vi "Receiver_Example - 2 Channel - Experiment_10.vi"() -> ()   [LabVIEW 2022 SP3]
uses:
  <vilib>/httpClient/LabVIEWHTTPClient.lvlib
panel:
  out "LP - CH0 3":dbl format="%#_4g"
  out "LP - CH0 2":dbl format="%#_4g"
  out "HP - CH0 3":dbl format="%#_4g"
  out "HP - CH0 2":dbl format="%#_4g"
  out ".not. x?":bool
  out "BER 16QAM":dbl
  out "LP - CH0":dbl format="%#_4g"
  in  "url 2":string="http://Cobot280-02.local:5000"
  out "Numeric":i32
  out "HP - CH0":dbl format="%#_4g"
  in  "url":string="http://Cobot280-01.local:5000"
  out "x = 0?":bool
  out "iterationsIM":dbl
  in  "State":i32
  in  "Counter":dbl
  in  "OFDM - 4QAM/16QAM":bool
  in  "Tab Control 3":enum32{"OFDM - 4QAM", "16QAM"}(tab)
  in  "Tab Control":enum32{"USRP Parameters", "Rx Info", "BER"}(tab)
  in  "USRP ControledParameters":T1={"Active Antenna"="RX2", "Gain (dB)"=10.0, "Carrier Frequency"=2400000000.0, "IQ Rate"=2000000.0, "Active channels"="0,1"} {"IQ Rate" format="%#_6p"; "Carrier Frequency" format="%#_6p"; "Gain (dB)" format="%#_6f"}
  in  "Device selection":refnum<k15>="RIO0"
  in  "Trigger level":dbl=0.005 format="%f"
  out "CH0":T2
  out "CH1":T2
  out "SIG valid? - CH1":bool
  out "SIG valid? - CH0":bool
  out "Frequency offset - CH1":dbl
  out "Frequency offset - CH0":dbl
  out "Coerced Parameters":T3={"IQ Rate"=100000.0, "Carrier  Freq."=100000.0, "Gain"=0.0} {"Gain" format="%#_6f"; "Carrier  Freq." format="%#_6p"; "IQ Rate" format="%#_6p"}
  out "Error out":errorcluster
  in  "Expected message LP - CH0":string="Non Critical Data\nNon Critical Data\nNon Critical Data\nNon Critical Data\nNon Critical Data"
  in  "Expected message - CH1":string="Critical Dataaaaa\nCritical Dataaaaa\nCritical Dataaaaa\nCritical Dataaaaa\nCritical Dataaaaa"
  out "Expected message LP Detected CH0":string="Non Critical Data\nNon Critical Data\nNon Critical Data\nNon Critical Data\nNon Critical Data"
  out "Expected message HP Detected CH1":string="Non Critical Data\nNon Critical Data\nNon Critical Data\nNon Critical Data\nNon Critical Data"
  in  "Boolean":bool
  in  "Boolean 3":bool
  out "Expected message HP Detected CH0":string="Non Critical Data\nNon Critical Data\nNon Critical Data\nNon Critical Data\nNon Critical Data"
  in  "Expected message HP - CH0":string="Critical Dataaaaa\nCritical Dataaaaa\nCritical Dataaaaa\nCritical Dataaaaa\nCritical Dataaaaa"
  in  "Boolean 2":bool
  out "Inst. BER HP - CH0":dbl format="%#_4g"
  out "Acc. BER HP - CH0":dbl format="%#_4g"
  out "Acum. Err HP - CH0":dbl
  out "No. Bits HP - CH0":dbl
  out "Acc. BER LP - CH0":dbl format="%#_4g"
  out "Inst. BER - CH1":dbl format="%#_4g"
  out "Inst. BER LP - CH0":dbl format="%#_4g"
  out "No. Bits - CH1":dbl
  out "No. Bits LP - CH0":dbl
  out "Acum. Err - CH1":dbl
  out "Acum. Err LP - CH0":dbl
  in  "Record BER":bool
  in  "Refresh Button":bool
  out "Acc. BER - CH1":dbl format="%#_4g"
  in  "Low-Power Window Size - CH0":dbl=15.0 format="%#_6p"
  in  "High-Power Window Size":dbl=15.0 format="%#_6p"
  in  "Tab Control 2":enum32{"1 Channel", "2 Channel"}(tab)
  in  "Save data 1 channel":bool
  out "Constellation Map 1 Channel":cdb[](graph)
  out "Low-Power BER - 1 Channel":dbl(graph)
  out "High-Power BER - 1 Channel":dbl(graph)
  out "High-Power Decoded message - 1 Channel":string
  out "Low-Power Decoded message - 1 Channel":string
  in  "Color Box":u32(colorbox)=11025761
  in  "Color Box 2":u32(colorbox)=7377308
  out "Low-Power Decoded message - CH0":string
  out "Decoded message - CH1":string
  out "Constellation Map 2 Channel":cluster{"Constellation":cdb[]}[](graph)
  out "Low-Power BER - CH0":dbl(graph)
  out "High-Power BER":T4(graph)
  out "High-Power Decoded message - CH0":string
  out "CH1 2":bool
  out "CH0 2":bool
  in  "Save data 2 channels":bool
  in  "Channel":bool
  in  "Threshold":dbl=10.0
  in  "Save data":bool
  out "Expected message  HP  Detected 2":string="Critical Dataaaaa\nCritical Dataaaaa\nCritical Dataaaaa\nCritical Dataaaaa\nCritical Dataaaaa"
  in  "Boolean 4":bool
  in  "High-Power Window Size 2":dbl=15.0 format="%#_6p"
  out "High-Power Instantaneous BER Graph 2":u8(slide) scale=0.0..100.0
  out "High-Power BER Graph 2":dbl(graph)
  out "No. Bits HP 2":dbl
  out "Acc. BER  HP 2":dbl format="%#_4g"
  out "Acum. Err HP 2":dbl
  out "Inst. BER HP 2":dbl format="%#_4g"
  in  "Expected message 2 HP 2":string="Critical Dataaaaa\nCritical Dataaaaa\nCritical Dataaaaa\nCritical Dataaaaa\nCritical Dataaaaa"
  out "High-Power Decoded Message 2":string
  in  "Record BER 2":bool
  out "Constellation Map 2":cdb[](graph)
  out "Frequency offset 2":dbl
  out "SIG valid? 2":bool
  in  "Refresh Button 2":bool
  out "Error out 2":errorcluster
  in  "error in (no error)":errorcluster
  # "OFDM Superposition Coded Receiver"
  # "1 Channel"
  # "2 Channel"
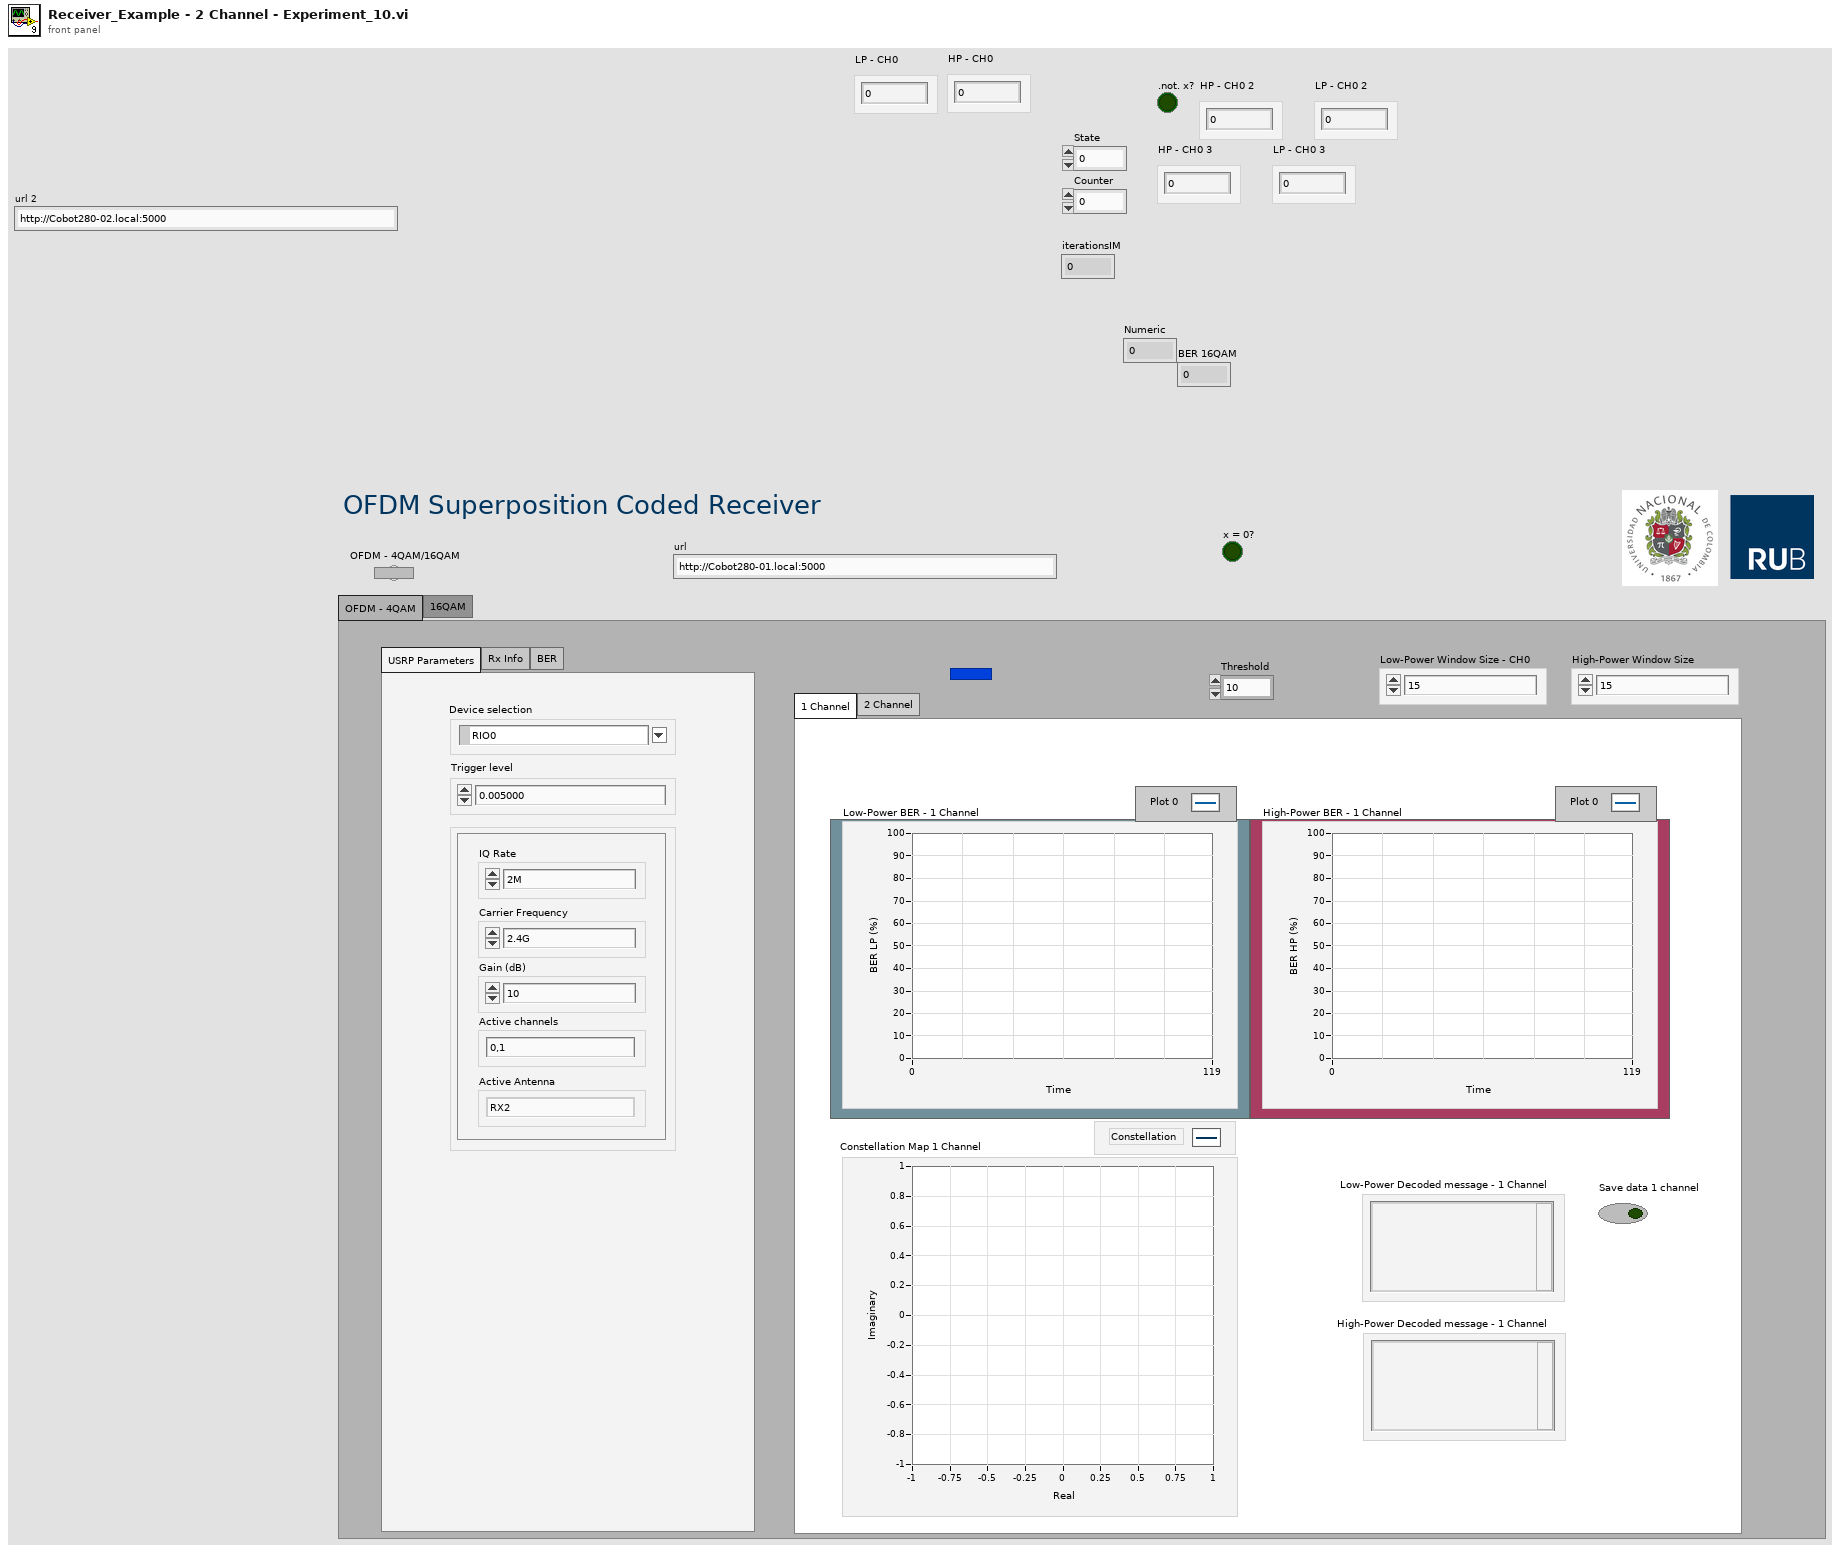
[diagram p1: front panel]
types:
  T1 = cluster{"Active Antenna":string, "Gain (dB)":dbl, "Carrier Frequency":dbl, "IQ Rate":dbl, "Active channels":string}
  T2 = cluster{"Modulation type":enum16{"QPSK(4QAM)", "64QAM", "16QAM", "BPSK"}, "BCC rate (k/n)":enum16{"1/2", "2/3", "3/4"}}
  T3 = cluster{"IQ Rate":dbl, "Carrier  Freq.":dbl, "Gain":dbl}
  T4 = cluster{"Graph Instantaneous BER":dbl, "Graph Instantaneous BER":dbl, "Inst. BER - CH1":dbl}
  T5 = enum16{"open", "replace", "create", "open or create", "replace or create", "replace or create with confirmation"}
  T6 = cluster{"coerced IQ rate":dbl, "coerced carrier frequency":dbl, "coerced gain":dbl}
  T7 = cluster{"Graph Instantaneous BER":dbl, "Graph Instantaneous BER":dbl, "Graph Instantaneous BER":dbl}
  T8 = typedef "LabVIEWHTTPClient.lvlib/ClientHandle.ctl" = refnum<k1>
  T9 = typedef "angle_speed_def.ctl" = cluster{"degrees":dbl[], "speed":i32}
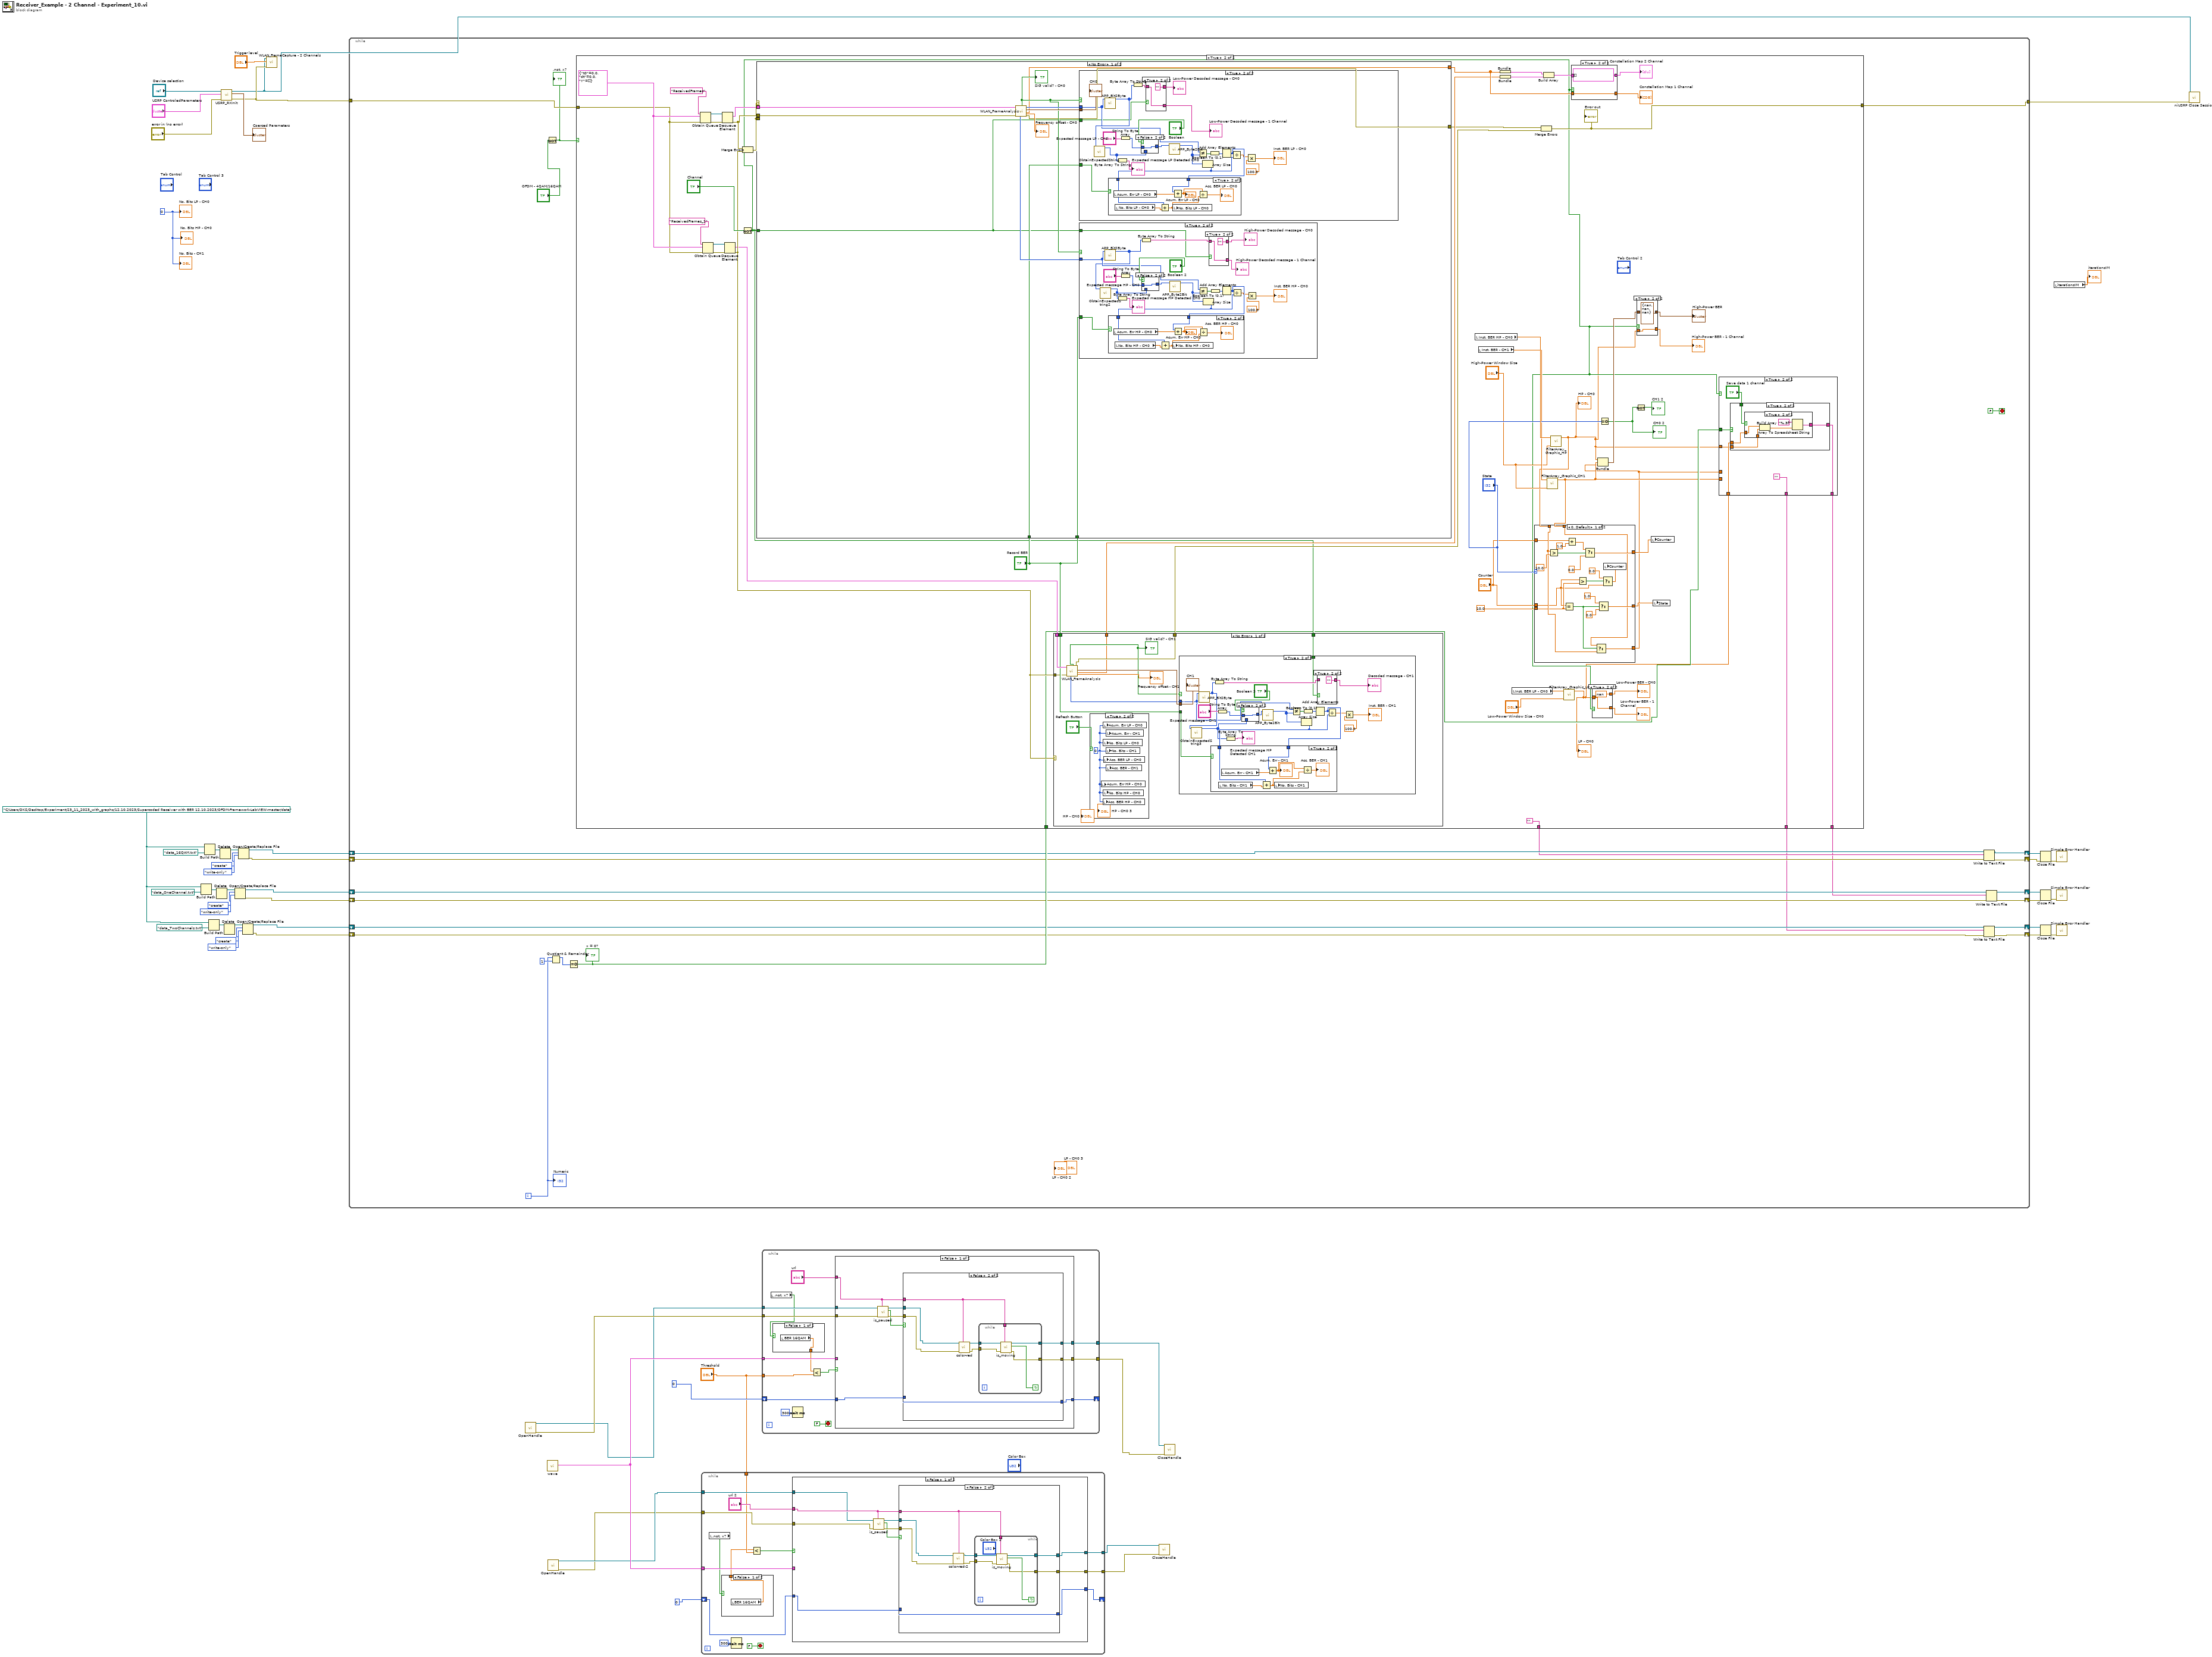
[diagram p0: block diagram]
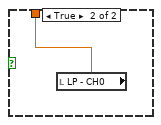
[diagram p2: hidden frame]
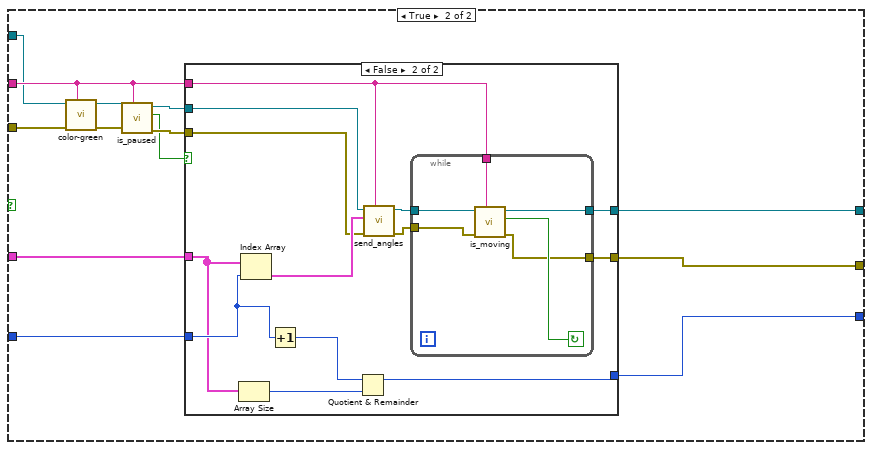
[diagram p4: hidden frame]
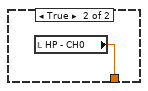
[diagram p6: hidden frame]
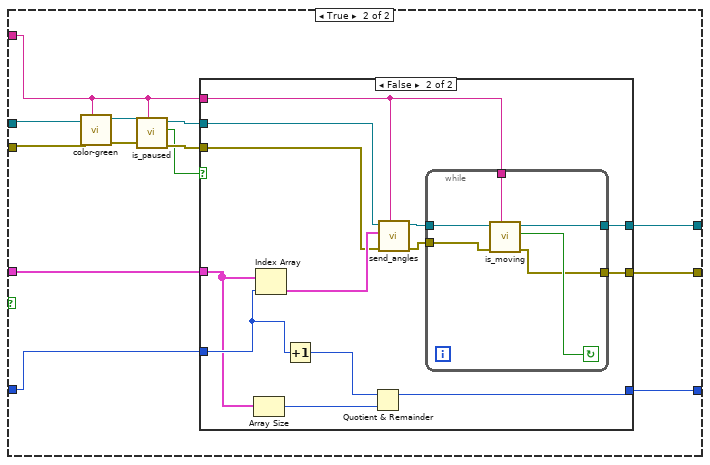
[diagram p8: hidden frame]
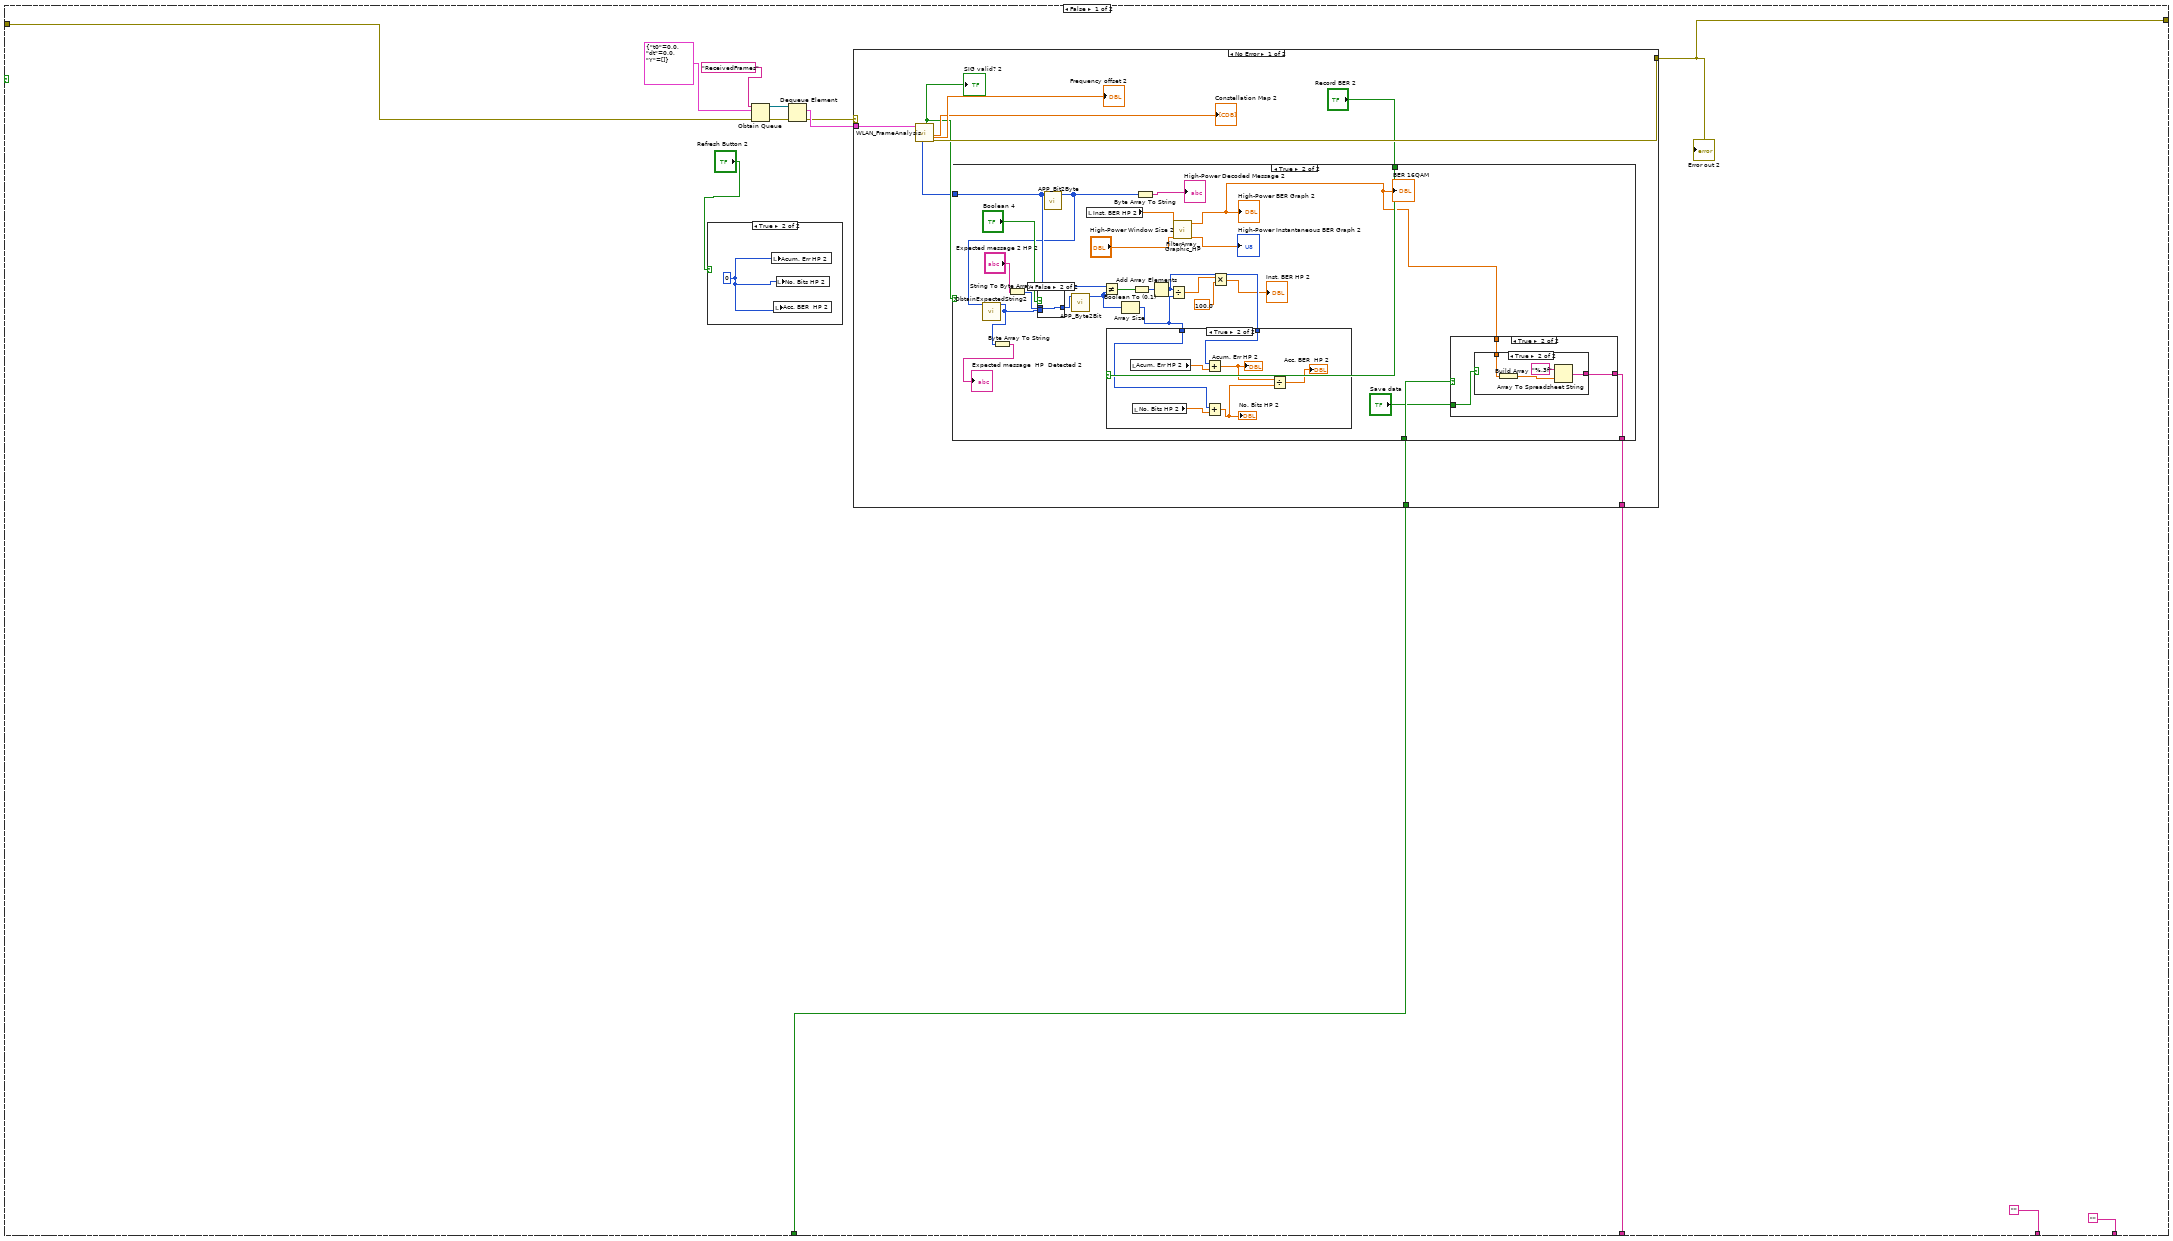
[diagram p10: hidden frame]
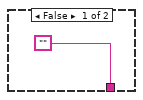
[diagram p12: hidden frame]
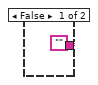
[diagram p13: hidden frame]
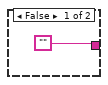
[diagram p14: hidden frame]
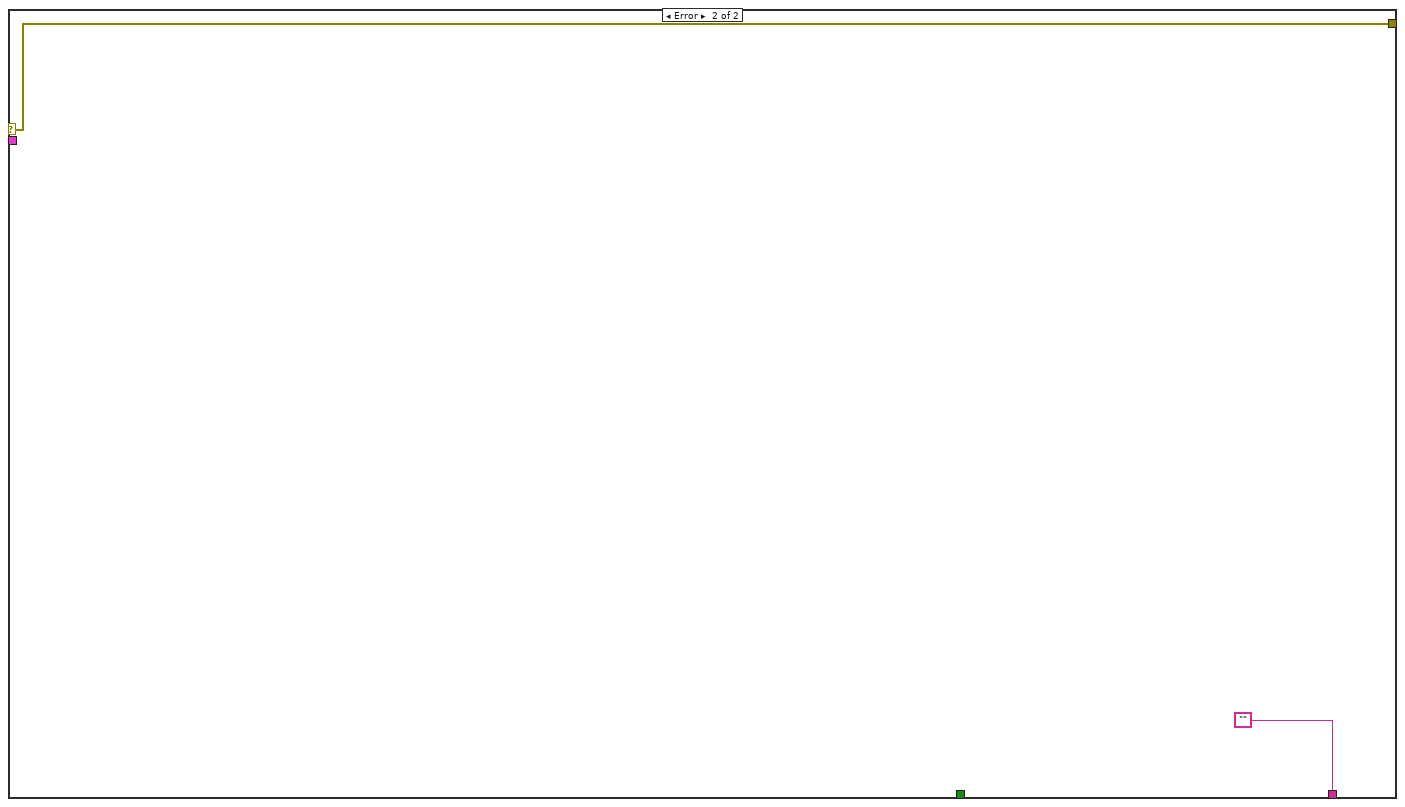
[diagram p17: hidden frame]
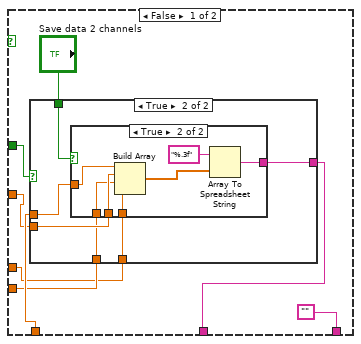
[diagram p18: hidden frame]
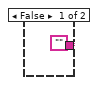
[diagram p19: hidden frame]
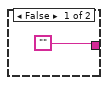
[diagram p20: hidden frame]
diagram:
  w23 = path "C:/Users/DKS/Desktop/Experiment/23_11_2023_with_graphs/12.10.2023/Supercoded Receiver with BER 12.10.2023/OFDM-Framework-LabVIEW-master/data"
  w45 = 0
  n1 = Build Path(base path=w23, name or relative path=path "data_OneChannel.txt" ("default name")) -> (appended path=w33:path)
  n2 = Build Path(base path=w23, name or relative path=path "data_16QAM.txt" ("default name")) -> (appended path=w43:path)
  n3 = Build Path(base path=w23, name or relative path=path "data_TwoChannels.txt" ("default name")) -> (appended path=w28:path)
  n4 = Delete(path (use dialog)=w33) -> (deleted path=w32:path)  [unwired: 4 in, 2 out]
  n5 = Delete(path (use dialog)=w43) -> (deleted path=w42:path)  [unwired: 4 in, 2 out]
  n6 = call "USRP_RXInit.vi"("device names"="Device selection", "USRP ControledParameters"="USRP ControledParameters", "error in (no error)"="error in (no error)") -> ("session handle out"=w48:refnum<k15>, "USRP CoercedParamters"=→"Coerced Parameters":T6, "error out"=w51:errorcluster)  [unwired: 5 in]
  n7 = Delete(path (use dialog)=w28) -> (deleted path=w27:path)  [unwired: 4 in, 2 out]
  n8 = Open/Create/Replace File(file path (use dialog)=w32, operation (0:open)=T5."create", access (0:read/write)=enum16{"read/write", "read-only", "write-only"}."write-only") -> (refnum out=w20:refnum<file>, error out=w19:errorcluster)  [unwired: 1 in, 3 out]
  n9 = Open/Create/Replace File(file path (use dialog)=w42, operation (0:open)=T5."create", access (0:read/write)=enum16{"read/write", "read-only", "write-only"}."write-only") -> (refnum out=w36:refnum<file>, error out=w37:errorcluster)  [unwired: 1 in, 3 out]
  n10 = Open/Create/Replace File(file path (use dialog)=w27, operation (0:open)=T5."create", access (0:read/write)=enum16{"read/write", "read-only", "write-only"}."write-only") -> (refnum out=w18:refnum<file>, error out=w17:errorcluster)  [unwired: 1 in, 3 out]
  n11 = call "WLAN_FrameCapture - 2 Channels.vi"("error in (no error)"=w51, "Trigger level"="Trigger level", "session handle"=w48) -> ()  [unwired: 8 in]
  n12 = while {
    tunnel: w51 -> [w77]
    tunnel: [w76] -> w49
    shift-right: [w69] -> w35
    shift-left: w37 -> [w67]
    shift-right: [w68] -> w34
    shift-left: w36 -> [w66]
    shift-right: [w63] -> w16
    shift-left: w20 -> [w64]
    shift-right: [w61] -> w15
    shift-left: w19 -> [w62]
    shift-right: [w57] -> w14
    shift-left: w18 -> [w60]
    shift-right: [w58] -> w13
    shift-left: w17 -> [w59]
    i -> [w54]
    stop <- FALSE stop-if-true
    n13 = Not(x="OFDM - 4QAM/16QAM") -> (.not. x?=w74:bool)
    ".not. x?" <- w74
    n14 = Quotient & Remainder(x=w54, y=1) -> (x-y*floor(x/y)=w71:i32)  [unwired: 1 out]
    n15 = Equal To 0?(x=w71) -> (x = 0?=w70:bool)
    "x = 0?" <- w70
    n16 = case shown="True" w74 {
      tunnel: w77 -> [w83 w161]
      tunnel: [w82 w160] -> w76
      tunnel: w70 -> [w81 w153]
      tunnel: [w80 ""] -> w65
      tunnel: ["" w152] -> w56
      tunnel: ["" w150] -> w55
      frame False {
        n17 = case shown="True" "Refresh Button 2" {
          frame False {
          }
          frame True {
            w91 = 0
            n18 = local write "Acum. Err HP 2"(w91) -> ()
            n19 = local write "Acc. BER  HP 2"(w91) -> ()
            n20 = local write "No. Bits HP 2"(w91) -> ()
          }
        }
        n21 = Obtain Queue(name (unnamed)="ReceivedFrames", element data type=cluster{"t0":dbl, "dt":dbl, "Y":cdb[]} {"t0"=0.0, "dt"=0.0, "Y"=[]} ("data"), error in (no error)=w83) -> (queue out=w84:refnum<queue>, error out=w87:errorcluster)  [unwired: 2 in, 1 out]
        n22 = Dequeue Element(queue=w84, error in (no error)=w87) -> (element=w86:cluster{"t0":dbl, "dt":dbl, "Y":cdb[]}, error out=w85:errorcluster)  [unwired: 1 in, 2 out]
        n23 = case shown="No Error" w85 {
          selector: w85 -> [_ w146]
          tunnel: w86 -> [w99 _]
          tunnel: [w100 w146] -> w82
          tunnel: w81 -> [w93 _]
          tunnel: [w92 ""] -> w80
          frame No Error {
            n24 = call "WLAN_FrameAnalysis.vi"("input cluster"=w99) -> ("error out"=w100:errorcluster, "Constellation"=→"Constellation Map 2":cdb[], "Frequency offset"=→"Frequency offset 2":dbl, "SIG valid?"=w95:bool, "outputbitsHP"=w94:i8[])  [unwired: 4 in, 2 out]
            "SIG valid? 2" <- w95
            n25 = case shown="True" w95 {
              tunnel: "Record BER 2" -> [_ w120]
              tunnel: w94 -> [_ w115]
              tunnel: w93 -> [_ w105]
              tunnel: ["" w103] -> w92
              frame False {
              }
              frame True {
                n26 = String To Byte Array(string="Expected message 2 HP 2") -> (unsigned byte array=w113:u8[])
                n27 = call "APP_Bit2Byte.vi"("input bit stream"=w115) -> ("output byte stream"=w109:u8[])  [unwired: 10 in]
                n28 = call "ObtainExpectedString2.vi"("Array"=w109) -> ("detectedMessage"=w111:i8[])  [unwired: 9 in]
                n29 = Byte Array To String(unsigned byte array=w111) -> (string=→"Expected message  HP  Detected 2":string)
                n30 = case shown="False" "Boolean 4" {
                  tunnel: [w136 w137] -> w114
                  tunnel: w113 -> [_ w137]
                  tunnel: w111 -> [w136 _]
                  frame True {
                  }
                  frame False {
                  }
                }
                n31 = call "APP_Byte2Bit.vi"("input byte stream"=w114) -> ("output bit stream"=w116:i8[])  [unwired: 10 in]
                n32 = local read "Inst. BER HP 2"() -> (w119:dbl)
                n33 = Not Equal?(x=w115, y=w116) -> (x != y?=w124:bool[])
                n34 = Array Size(array=w116) -> (size(s)=w121:i32)
                n35 = Boolean To (0,1)(Boolean=w124) -> (0, 1=w123:i16[])
                n36 = Byte Array To String(unsigned byte array=w109) -> (string=→"High-Power Decoded Message 2":string)
                n37 = Add Array Elements(numeric array=w123) -> (sum=w122:i16)
                n38 = case shown="True" w120 {
                  tunnel: w122 -> [_ w143]
                  tunnel: w121 -> [_ w138]
                  frame False {
                  }
                  frame True {
                    n39 = local read "Acum. Err HP 2"() -> (w144:dbl)
                    n40 = local read "No. Bits HP 2"() -> (w140:dbl)
                    n41 = Add(x=w143, y=w144) -> (x+y=w142:dbl)
                    "Acum. Err HP 2" <- w142
                    n42 = Add(x=w138, y=w140) -> (x+y=w139:dbl)
                    "No. Bits HP 2" <- w139
                    n43 = Divide(x=w142, y=w139) -> (x/y=→"Acc. BER  HP 2":dbl)
                  }
                }
                n44 = Divide(x=w122, y=w121) -> (x/y=w108:dbl)
                n45 = call "FilterArray_Graphic_HP.vi"("Window Size"="High-Power Window Size 2", "Instantaneous BER"=w119) -> ("Slide Bar"=→"High-Power Instantaneous BER Graph 2":dbl, "Graph Instantaneous BER"=w102:dbl)  [unwired: 4 in]
                "High-Power BER Graph 2" <- w102
                "BER 16QAM" <- w102
                n46 = Multiply(x=w108, y=100.0) -> (x*y=→"Inst. BER HP 2":dbl)
                n47 = case shown="True" w105 {
                  tunnel: ["" w130] -> w103
                  tunnel: w102 -> [_ w129]
                  tunnel: "Save data" -> [_ w128]
                  frame False {
                  }
                  frame True {
                    n48 = case shown="True" w128 {
                      tunnel: ["" w133] -> w130
                      tunnel: w129 -> [_ w132]
                      frame False {
                      }
                      frame True {
                        n49 = Build Array(w132) -> (w135:dbl[])
                        n50 = Array To Spreadsheet String(array=w135, 3:"%.3f") -> (spreadsheet string=w133:string)  [unwired: 1 out]
                      }
                    }
                  }
                }
              }
            }
          }
          frame Error {
          }
        }
        "Error out 2" <- w82
      }
      frame True {
        w197 = cluster{"t0":dbl, "dt":dbl, "Y":cdb[]} {"t0"=0.0, "dt"=0.0, "Y"=[]} ("data")
        n51 = Obtain Queue(name (unnamed)="ReceivedFrames", element data type=w197, error in (no error)=w161) -> (queue out=w162:refnum<queue>, error out=w164:errorcluster)  [unwired: 2 in, 1 out]
        n52 = Obtain Queue(name (unnamed)="ReceivedFrames_1", element data type=w197, error in (no error)=w161) -> (queue out=w166:refnum<queue>, error out=w167:errorcluster)  [unwired: 2 in, 1 out]
        n53 = Dequeue Element(queue=w162, error in (no error)=w164) -> (element=w163:cluster{"t0":dbl, "dt":dbl, "Y":cdb[]}, error out=w170:errorcluster)  [unwired: 1 in, 2 out]
        n54 = Dequeue Element(queue=w166, error in (no error)=w167) -> (element=w172:cluster{"t0":dbl, "dt":dbl, "Y":cdb[]}, error out=w176:errorcluster)  [unwired: 1 in, 2 out]
        n55 = Not(x="Channel") -> (.not. x?=w154:bool)
        n56 = Merge Errors(w170, w176) -> (w169:errorcluster)
        n57 = case shown="No Error" w169 {
          tunnel: w163 -> [w342 _]
          tunnel: w169 -> [_ w416]
          tunnel: w170 -> [w339 _]
          tunnel: [w338 dbl[] []] -> w188
          tunnel: [w337 w416] -> w173
          tunnel: "Record BER" -> [w336 _]
          tunnel: "Record BER" -> [w335 _]
          tunnel: w154 -> [w334 _]
          frame No Error {
            n58 = call "WLAN_FrameAnalysis.vi"("error in (no error)"=w339, "input cluster"=w342) -> ("error out"=w337:errorcluster, "Constellation"=w338:cdb[], "Modulation parameter"=w343:T2, "output bits"=w344:i8[], "Frequency offset"=→"Frequency offset - CH0":dbl, "SIG valid?"=w340:bool, "outputbitsHP"=w341:i8[])  [unwired: 3 in]
            "SIG valid? - CH0" <- w340
            n59 = case shown="True" w340 {
              tunnel: w344 -> [_ w385]
              tunnel: w343 -> [_ w401]
              tunnel: w335 -> [_ w397]
              tunnel: w334 -> [_ w380]
              frame False {
              }
              frame True {
                n60 = call "APP_Bit2Byte.vi"("input bit stream"=w385) -> ("output byte stream"=w389:u8[])  [unwired: 10 in]
                n61 = call "ObtainExpectedString.vi"("Array"=w389) -> ("detectedMessage"=w386:i8[])  [unwired: 9 in]
                n62 = Byte Array To String(unsigned byte array=w386) -> (string=→"Expected message LP Detected CH0":string)
                n63 = String To Byte Array(string="Expected message LP - CH0") -> (unsigned byte array=w390:u8[])
                n64 = Byte Array To String(unsigned byte array=w389) -> (string=w383:string)
                n65 = case shown="False" "Boolean" {
                  tunnel: [w406 w407] -> w392
                  tunnel: w390 -> [_ w407]
                  tunnel: w386 -> [w406 _]
                  frame True {
                  }
                  frame False {
                  }
                }
                n66 = case shown="True" w380 {
                  tunnel: w383 -> [w403 w405]
                  tunnel: ["" ("string") w405] -> w382
                  tunnel: [w403 "" ("string")] -> w381
                  frame False {
                  }
                  frame True {
                  }
                }
                "Low-Power Decoded message - CH0" <- w381
                "Low-Power Decoded message - 1 Channel" <- w382
                n67 = call "APP_Byte2Bit.vi"("input byte stream"=w392) -> ("output bit stream"=w391:i8[])  [unwired: 10 in]
                n68 = Not Equal?(x=w385, y=w391) -> (x != y?=w399:bool[])
                n69 = Array Size(array=w391) -> (size(s)=w396:i32)
                n70 = Boolean To (0,1)(Boolean=w399) -> (0, 1=w400:i16[])
                n71 = Add Array Elements(numeric array=w400) -> (sum=w395:i16)
                n72 = case shown="True" w397 {
                  tunnel: w396 -> [_ w413]
                  tunnel: w395 -> [_ w411]
                  frame False {
                  }
                  frame True {
                    n73 = local read "Acum. Err LP - CH0"() -> (w412:dbl)
                    n74 = local read "No. Bits LP - CH0"() -> (w414:dbl)
                    n75 = Add(x=w413, y=w414) -> (x+y=w410:dbl)
                    n76 = Add(x=w411, y=w412) -> (x+y=w409:dbl)
                    "Acum. Err LP - CH0" <- w409
                    n77 = local write "No. Bits LP - CH0"(w410) -> ()
                    n78 = Divide(x=w409, y=w410) -> (x/y=→"Acc. BER LP - CH0":dbl)
                  }
                }
                n79 = Divide(x=w395, y=w396) -> (x/y=w394:dbl)
                n80 = Multiply(x=w394, y=100.0) -> (x*y=→"Inst. BER LP - CH0":dbl)
                "CH0" <- w401
              }
            }
            n81 = case shown="True" w340 {
              tunnel: w341 -> [_ w353]
              tunnel: w336 -> [_ w363]
              tunnel: w334 -> [_ w346]
              frame False {
              }
              frame True {
                n82 = call "APP_Bit2Byte.vi"("input bit stream"=w353) -> ("output byte stream"=w352:u8[])  [unwired: 10 in]
                n83 = call "ObtainExpectedString2.vi"("Array"=w352) -> ("detectedMessage"=w351:i8[])  [unwired: 9 in]
                n84 = Byte Array To String(unsigned byte array=w351) -> (string=→"Expected message HP Detected CH0":string)
                n85 = String To Byte Array(string="Expected message HP - CH0") -> (unsigned byte array=w356:u8[])
                n86 = Byte Array To String(unsigned byte array=w352) -> (string=w347:string)
                n87 = case shown="False" "Boolean 2" {
                  tunnel: [w371 w372] -> w358
                  tunnel: w356 -> [_ w372]
                  tunnel: w351 -> [w371 _]
                  frame True {
                  }
                  frame False {
                  }
                }
                n88 = call "APP_Byte2Bit.vi"("input byte stream"=w358) -> ("output bit stream"=w357:i8[])  [unwired: 10 in]
                n89 = Not Equal?(x=w353, y=w357) -> (x != y?=w365:bool[])
                n90 = Array Size(array=w357) -> (size(s)=w362:i32)
                n91 = case shown="True" w346 {
                  tunnel: w347 -> [w368 w370]
                  tunnel: ["" ("string") w370] -> w348
                  tunnel: [w368 "" ("string")] -> w349
                  frame False {
                  }
                  frame True {
                  }
                }
                "High-Power Decoded message - CH0" <- w349
                "High-Power Decoded message - 1 Channel" <- w348
                n92 = Boolean To (0,1)(Boolean=w365) -> (0, 1=w366:i16[])
                n93 = Add Array Elements(numeric array=w366) -> (sum=w361:i16)
                n94 = case shown="True" w363 {
                  tunnel: w362 -> [_ w378]
                  tunnel: w361 -> [_ w376]
                  frame False {
                  }
                  frame True {
                    n95 = local read "Acum. Err HP - CH0"() -> (w377:dbl)
                    n96 = local read "No. Bits HP - CH0"() -> (w379:dbl)
                    n97 = Add(x=w378, y=w379) -> (x+y=w375:dbl)
                    n98 = local write "No. Bits HP - CH0"(w375) -> ()
                    n99 = Add(x=w376, y=w377) -> (x+y=w374:dbl)
                    "Acum. Err HP - CH0" <- w374
                    n100 = Divide(x=w374, y=w375) -> (x/y=→"Acc. BER HP - CH0":dbl)
                  }
                }
                n101 = Divide(x=w361, y=w362) -> (x/y=w360:dbl)
                n102 = Multiply(x=w360, y=100.0) -> (x*y=→"Inst. BER HP - CH0":dbl)
              }
            }
          }
          frame Error {
          }
        }
        n103 = case shown="No Error" w176 {
          tunnel: w172 -> [w294 _]
          tunnel: "Record BER" -> [w292 _]
          tunnel: [w291 w333] -> w174
          tunnel: [w290 dbl[] []] -> w175
          tunnel: w176 -> [w289 w333]
          tunnel: w154 -> [w288 _]
          frame No Error {
            n104 = call "WLAN_FrameAnalysis.vi"("error in (no error)"=w289, "input cluster"=w294) -> ("error out"=w291:errorcluster, "Constellation"=w290:cdb[], "Modulation parameter"=w297:T2, "Frequency offset"=→"Frequency offset - CH1":dbl, "SIG valid?"=w293:bool, "outputbitsHP"=w295:i8[])  [unwired: 3 in, 1 out]
            "SIG valid? - CH1" <- w293
            n105 = case shown="True" "Refresh Button" {
              frame False {
              }
              frame True {
                w299 = 0
                n106 = local write "Acum. Err HP - CH0"(w299) -> ()
                n107 = local write "Acc. BER HP - CH0"(w299) -> ()
                n108 = local write "Acum. Err LP - CH0"(w299) -> ()
                n109 = local write "No. Bits LP - CH0"(w299) -> ()
                n110 = local write "No. Bits HP - CH0"(w299) -> ()
                n111 = local write "Acc. BER LP - CH0"(w299) -> ()
                n112 = local write "Acum. Err - CH1"(w299) -> ()
                n113 = local write "No. Bits - CH1"(w299) -> ()
                n114 = local write "Acc. BER - CH1"(w299) -> ()
              }
            }
            n115 = case shown="True" w293 {
              tunnel: w295 -> [_ w306]
              tunnel: w297 -> [_ w320]
              tunnel: w292 -> [_ w303]
              tunnel: w288 -> [_ w300]
              frame False {
              }
              frame True {
                n116 = call "APP_Bit2Byte.vi"("input bit stream"=w306) -> ("output byte stream"=w309:u8[])  [unwired: 10 in]
                n117 = call "ObtainExpectedString3.vi"("Array"=w309) -> ("detectedMessage"=w308:i8[])  [unwired: 9 in]
                n118 = Byte Array To String(unsigned byte array=w309) -> (string=w301:string)
                n119 = String To Byte Array(string="Expected message - CH1") -> (unsigned byte array=w310:u8[])
                n120 = Byte Array To String(unsigned byte array=w308) -> (string=→"Expected message HP Detected CH1":string)
                n121 = case shown="False" "Boolean 3" {
                  tunnel: [w323 w324] -> w312
                  tunnel: w310 -> [_ w324]
                  tunnel: w308 -> [w323 _]
                  frame True {
                  }
                  frame False {
                  }
                }
                n122 = call "APP_Byte2Bit.vi"("input byte stream"=w312) -> ("output bit stream"=w311:i8[])  [unwired: 10 in]
                n123 = Not Equal?(x=w306, y=w311) -> (x != y?=w318:bool[])
                n124 = Array Size(array=w311) -> (size(s)=w316:i32)
                n125 = Boolean To (0,1)(Boolean=w318) -> (0, 1=w319:i16[])
                n126 = Add Array Elements(numeric array=w319) -> (sum=w315:i16)
                n127 = case shown="True" w303 {
                  tunnel: w316 -> [_ w330]
                  tunnel: w315 -> [_ w328]
                  frame False {
                  }
                  frame True {
                    n128 = local read "No. Bits - CH1"() -> (w331:dbl)
                    n129 = local read "Acum. Err - CH1"() -> (w329:dbl)
                    n130 = Add(x=w330, y=w331) -> (x+y=w327:dbl)
                    n131 = Add(x=w328, y=w329) -> (x+y=w326:dbl)
                    "Acum. Err - CH1" <- w326
                    n132 = local write "No. Bits - CH1"(w327) -> ()
                    n133 = Divide(x=w326, y=w327) -> (x/y=→"Acc. BER - CH1":dbl)
                  }
                }
                n134 = case shown="True" w300 {
                  tunnel: w301 -> [w321 _]
                  tunnel: [w321 "" ("string")] -> w302
                  frame False {
                  }
                  frame True {
                  }
                }
                "Decoded message - CH1" <- w302
                n135 = Divide(x=w315, y=w316) -> (x/y=w313:dbl)
                n136 = Multiply(x=w313, y=100.0) -> (x*y=→"Inst. BER - CH1":dbl)
                "CH1" <- w320
              }
            }
          }
          frame Error {
          }
        }
        n137 = local read "Inst. BER HP - CH0"() -> (w193:dbl)
        n138 = local read "Inst. BER - CH1"() -> (w183:dbl)
        n139 = Bundle("Constellation"=w188) -> (w187:cluster{"Constellation":cdb[]})  [unwired: 1 in]
        n140 = Bundle("Constellation"=w175) -> (w171:cluster{"Constellation":cdb[]})  [unwired: 1 in]
        n141 = local read "Inst. BER LP - CH0"() -> (w156:dbl)
        n142 = Merge Errors(w173, w174) -> (w160:errorcluster)
        "Error out" <- w160
        n143 = Build Array(w187, w171) -> (w190:cluster{"Constellation":cdb[]}[])
        n144 = call "FilterArray_Graphic_CH1.vi"("Window Size"="High-Power Window Size", "Instantaneous BER"=w183) -> ("Graph Instantaneous BER"=w151:dbl)  [unwired: 4 in, 1 out]
        n145 = call "FilterArray_Graphic_HP.vi"("Window Size"="High-Power Window Size", "Instantaneous BER"=w193) -> ("Graph Instantaneous BER"=w148:dbl)  [unwired: 4 in, 1 out]
        "HP - CH0" <- w148
        n146 = case shown="0, Default" "State" {
          tunnel: "Counter" -> [w256 w276]
          tunnel: [w263 w279] -> w179
          tunnel: "Counter" -> [w251 w269]
          tunnel: [w260 w278] -> w180
          tunnel: [w258 w277] -> w149
          tunnel: w148 -> [w257 w274]
          tunnel: w151 -> [w255 w275]
          tunnel: 10.0 ("y") -> [w254 w270]
          frame 0, Default {
            n147 = Greater?(x=w257, y=10.0) -> (0:w264:bool)
            n148 = Equal?(x=w251, y=w254) -> (x = y?=w259:bool)
            n149 = Add(x=w256, y=1.0) -> (x+y=w266:dbl)
            n150 = Greater?(x=w251, y=w254) -> (0:w253:bool)
            n151 = Select(t=w266, s=w264, f=0.0) -> (s? t:f=w263:dbl)
            n152 = Select(t=w255, s=w259, f=w257) -> (s? t:f=w258:dbl)
            n153 = Select(t=1.0, s=w259, f=0.0) -> (s? t:f=w260:dbl)
            n154 = Select(t=0.0, s=w253, f=w251) -> (s? t:f=w250:dbl)
            n155 = local write "Counter"(w250) -> ()
          }
          frame 1 {
            n156 = Less?(x=w274, y=10.0) -> (x < y?=w280:bool)
            n157 = Greater?(x=w269, y=w270) -> (0:w272:bool)
            n158 = Equal?(x=w269, y=w270) -> (x = y?=w282:bool)
            n159 = Add(x=w276, y=1.0) -> (x+y=w286:dbl)
            n160 = Select(t=w286, s=w280, f=0.0) -> (s? t:f=w279:dbl)
            n161 = Select(t=0.0, s=w272, f=w269) -> (s? t:f=w273:dbl)
            n162 = local write "Counter"(w273) -> ()
            n163 = Select(t=w274, s=w282, f=w275) -> (s? t:f=w277:dbl)
            n164 = Select(t=0.0, s=w282, f=1.0) -> (s? t:f=w278:dbl)
          }
        }
        n165 = call "FilterArray_Graphic_LP.vi"("Window Size"="Low-Power Window Size - CH0", "Instantaneous BER"=w156) -> ("Graph Instantaneous BER"=w147:dbl)  [unwired: 4 in, 1 out]
        "LP - CH0" <- w147
        n166 = case shown="True" w154 {
          tunnel: [cdb[] [] ("Constellation") w249] -> w189
          tunnel: w188 -> [_ w249]
          tunnel: w190 -> [w247 _]
          tunnel: [w247 cluster{"Constellation":cdb[]}[] []] -> w191
          frame False {
          }
          frame True {
          }
        }
        "Constellation Map 2 Channel" <- w191
        "Constellation Map 1 Channel" <- w189
        n167 = case shown="True" w154 {
          tunnel: w147 -> [w239 w241]
          tunnel: [nan ("Graph Instantaneous BER") w241] -> w157
          tunnel: [w239 nan ("Graph Instantaneous BER")] -> w158
          frame False {
          }
          frame True {
          }
        }
        "Low-Power BER - CH0" <- w158
        "Low-Power BER - 1 Channel" <- w157
        n168 = Bundle("Graph Instantaneous BER"=w148, "Graph Instantaneous BER"=w151, "Graph Instantaneous BER"=w149) -> (w195:T7)  [unwired: 1 in]
        n169 = Equal To 0?(x="State") -> (x = 0?=w186:bool)
        "CH0 2" <- w186
        n170 = Not(x=w186) -> (.not. x?=→"CH1 2":bool)
        n171 = case shown="True" w154 {
          tunnel: w148 -> [_ w245]
          tunnel: [nan w245] -> w194
          tunnel: w195 -> [w243 _]
          tunnel: [w243 T7 {"Graph Instantaneous BER"=nan, "Graph Instantaneous BER"=nan, "Graph Instantaneous BER"=nan}] -> w196
          frame False {
          }
          frame True {
          }
        }
        "High-Power BER" <- w196
        "High-Power BER - 1 Channel" <- w194
        n172 = local write "Counter"(w179) -> ()
        n173 = local write "State"(w180) -> ()
        n174 = case shown="True" w154 {
          tunnel: w147 -> [w202 w226]
          tunnel: w148 -> [w201 w225]
          tunnel: w153 -> [w204 w224]
          tunnel: ["" w222] -> w152
          tunnel: w151 -> [w200 _]
          tunnel: w149 -> [w199 _]
          tunnel: [w198 ""] -> w150
          frame False {
            n175 = case shown="True" w204 {
              tunnel: ["" w212] -> w198
              tunnel: w202 -> [_ w210]
              tunnel: w201 -> [_ w211]
              tunnel: "Save data 2 channels" -> [_ w209]
              tunnel: w200 -> [_ w208]
              tunnel: w199 -> [_ w207]
              frame False {
              }
              frame True {
                n176 = case shown="True" w209 {
                  tunnel: ["" w218] -> w212
                  tunnel: w210 -> [_ w217]
                  tunnel: w211 -> [_ w216]
                  tunnel: w208 -> [_ w215]
                  tunnel: w207 -> [_ w214]
                  frame False {
                  }
                  frame True {
                    n177 = Build Array(w217, w216, w215, w214) -> (w220:dbl[])
                    n178 = Array To Spreadsheet String(array=w220, 3:"%.3f") -> (spreadsheet string=w218:string)  [unwired: 1 out]
                  }
                }
              }
            }
          }
          frame True {
            n179 = case shown="True" w224 {
              tunnel: ["" w231] -> w222
              tunnel: w226 -> [_ w229]
              tunnel: w225 -> [_ w230]
              tunnel: "Save data 1 channel" -> [_ w228]
              frame False {
              }
              frame True {
                n180 = case shown="True" w228 {
                  tunnel: ["" w235] -> w231
                  tunnel: w229 -> [_ w234]
                  tunnel: w230 -> [_ w233]
                  frame False {
                  }
                  frame True {
                    n181 = Build Array(w234, w233) -> (w237:dbl[])
                    n182 = Array To Spreadsheet String(array=w237, 3:"%.3f") -> (spreadsheet string=w235:string)  [unwired: 1 out]
                  }
                }
              }
            }
          }
        }
      }
    }
    n183 = Write to Text File(file (use dialog)=w60, text=w55, error in=w59) -> (refnum out=w57:refnum<file>, error out=w58:errorcluster)  [unwired: 1 in, 1 out]
    n184 = Write to Text File(file (use dialog)=w66, text=w65, error in=w67) -> (refnum out=w68:refnum<file>, error out=w69:errorcluster)  [unwired: 1 in, 1 out]
    n185 = Write to Text File(file (use dialog)=w64, text=w56, error in=w62) -> (refnum out=w63:refnum<file>, error out=w61:errorcluster)  [unwired: 1 in, 1 out]
    "Numeric" <- w54
  }
  n186 = call <vilib>:"OpenHandle.vi"() -> ("client handle out"=w7:T8, "error out"=w8:errorcluster)  [unwired: 14 in]
  n187 = call "wave.vi"() -> ("sequenz"=w9:T9[])  [unwired: 11 in]
  n188 = call <vilib>:"OpenHandle.vi"() -> ("client handle out"=w3:T8, "error out"=w2:errorcluster)  [unwired: 14 in]
  n189 = while {
    shift-right: [w425] -> _
    shift-left: 0 -> [w426]
    tunnel: w9 -> [w424]
    tunnel: w2 -> [w423]
    tunnel: w3 -> [w422]
    tunnel: [w421] -> w6
    tunnel: [w420] -> w4
    tunnel: "Threshold" -> [w419]
    stop <- FALSE stop-if-true
    n190 = local read ".not. x?"() -> (w417:bool)
    n191 = case shown="False" w417 {
      tunnel: [w431 w432] -> w418
      frame False {
        n192 = local read "BER 16QAM"() -> (w431:dbl)
      }
      frame True {
        n193 = local read "LP - CH0"() -> (w432:dbl)
      }
    }
    n194 = Wait (ms)(milliseconds to wait=u32 300) -> ()  [unwired: 1 out]
    n195 = Less?(x=w418, y=w419) -> (x < y?=w428:bool)
    n196 = case shown="False" w428 {
      tunnel: "url 2" -> [w437 w467]
      tunnel: w426 -> [w439 w466]
      tunnel: [w438 w465] -> w425
      tunnel: w424 -> [_ w464]
      tunnel: w423 -> [w434 w463]
      tunnel: w422 -> [w433 w462]
      tunnel: [w436 w461] -> w421
      tunnel: [w435 w460] -> w420
      frame False {
        n197 = call "is_paused.vi"("url"=w437, "error in (no error)"=w434, "client handle"=w433) -> ("error out"=w441:errorcluster, "paused"=w440:bool, "client handle out"=w442:T8)  [unwired: 6 in]
        n198 = case shown="False" w440 {
          tunnel: w437 -> [_ w448]
          tunnel: w441 -> [w444 w450]
          tunnel: w442 -> [w445 w449]
          tunnel: [w445 w453] -> w436
          tunnel: [w444 w452] -> w435
          tunnel: w439 -> [w443 w451]
          tunnel: [w443 w451] -> w438
          frame True {
          }
          frame False {
            n199 = call "color-red-2.vi"("url"=w448, "error in (no error)"=w450, "client handle"=w449) -> ("error out"=w446:errorcluster, "client handle out"=w447:T8)  [unwired: 7 in]
            n200 = while {
              tunnel: w448 -> [w459]
              tunnel: w447 -> [w458]
              tunnel: w446 -> [w457]
              tunnel: [w455] -> w453
              tunnel: [w454] -> w452
              stop <- w456 continue-if-true
              n201 = call "is_moving.vi"("string"=w459, "error in (no error)"=w457, "client handle"=w458) -> ("error out"=w454:errorcluster, "moving"=w456:bool, "client handle out"=w455:T8)  [unwired: 6 in]
            }
          }
        }
      }
      frame True {
        n202 = call "color-green.vi"("url"=w467, "error in (no error)"=w463, "client handle"=w462) -> ("error out"=w469:errorcluster, "client handle out"=w468:T8)  [unwired: 7 in]
        n203 = call "is_paused.vi"("url"=w467, "error in (no error)"=w469, "client handle"=w468) -> ("error out"=w471:errorcluster, "paused"=w470:bool, "client handle out"=w472:T8)  [unwired: 6 in]
        n204 = case shown="False" w470 {
          tunnel: w464 -> [_ w480]
          tunnel: w466 -> [w473 w482]
          tunnel: w467 -> [_ w485]
          tunnel: w471 -> [w474 w487]
          tunnel: w472 -> [w475 w486]
          tunnel: [w473 w478] -> w465
          tunnel: [w475 w477] -> w461
          tunnel: [w474 w476] -> w460
          frame True {
          }
          frame False {
            n205 = Array Size(array=w480) -> (size(s)=w479:i32)
            n206 = Index Array(array=w480, index=w482) -> (element=w488:T9)
            n207 = Increment(x=w482) -> (x+1=w481:i32)
            n208 = Quotient & Remainder(x=w481, y=w479) -> (x-y*floor(x/y)=w478:i32)  [unwired: 1 out]
            n209 = call "send_angles.vi"("url"=w485, "error in (no error)"=w487, "angles and speed"=w488, "client handle"=w486) -> ("error out"=w483:errorcluster, "client handle out"=w484:T8)  [unwired: 6 in]
            n210 = while {
              tunnel: w485 -> [w494]
              tunnel: w484 -> [w493]
              tunnel: w483 -> [w492]
              tunnel: [w490] -> w477
              tunnel: [w489] -> w476
              stop <- w491 continue-if-true
              n211 = call "is_moving.vi"("string"=w494, "error in (no error)"=w492, "client handle"=w493) -> ("error out"=w489:errorcluster, "moving"=w491:bool, "client handle out"=w490:T8)  [unwired: 6 in]
            }
          }
        }
      }
    }
  }
  n212 = while {
    tunnel: w9 -> [w508]
    tunnel: w8 -> [w507]
    tunnel: w7 -> [w506]
    tunnel: [w505] -> w12
    tunnel: [w504] -> w5
    shift-right: [w502] -> _
    shift-left: 0 -> [w503]
    tunnel: "Threshold" -> [w497]
    stop <- FALSE stop-if-true
    n213 = local read ".not. x?"() -> (w495:bool)
    n214 = case shown="False" w495 {
      tunnel: [w509 w510] -> w496
      frame False {
        n215 = local read "BER 16QAM"() -> (w509:dbl)
      }
      frame True {
        n216 = local read "HP - CH0"() -> (w510:dbl)
      }
    }
    n217 = Wait (ms)(milliseconds to wait=u32 300) -> ()  [unwired: 1 out]
    n218 = Less?(x=w496, y=w497) -> (x < y?=w500:bool)
    n219 = case shown="False" w500 {
      tunnel: w508 -> [_ w548]
      tunnel: w503 -> [w515 w539]
      tunnel: w507 -> [w516 w540]
      tunnel: w506 -> [w517 w541]
      tunnel: [w513 w547] -> w505
      tunnel: [w512 w546] -> w504
      tunnel: [w514 w544] -> w502
      tunnel: "url" -> [w511 w538]
      frame False {
        n220 = call "is_paused.vi"("url"=w511, "error in (no error)"=w516, "client handle"=w517) -> ("error out"=w519:errorcluster, "paused"=w518:bool, "client handle out"=w520:T8)  [unwired: 6 in]
        n221 = case shown="False" w518 {
          tunnel: w511 -> [_ w524]
          tunnel: w519 -> [w522 w526]
          tunnel: w520 -> [w523 w525]
          tunnel: [w523 w531] -> w513
          tunnel: [w522 w530] -> w512
          tunnel: w515 -> [w521 w529]
          tunnel: [w521 w529] -> w514
          frame True {
          }
          frame False {
            n222 = call "color-red.vi"("url"=w524, "error in (no error)"=w526, "client handle"=w525) -> ("error out"=w527:errorcluster, "client handle out"=w528:T8)  [unwired: 7 in]
            n223 = while {
              tunnel: w524 -> [w537]
              tunnel: w528 -> [w536]
              tunnel: w527 -> [w535]
              tunnel: [w533] -> w531
              tunnel: [w532] -> w530
              stop <- w534 continue-if-true
              n224 = call "is_moving.vi"("string"=w537, "error in (no error)"=w535, "client handle"=w536) -> ("error out"=w532:errorcluster, "moving"=w534:bool, "client handle out"=w533:T8)  [unwired: 6 in]
            }
          }
        }
      }
      frame True {
        n225 = call "color-green.vi"("url"=w538, "error in (no error)"=w540, "client handle"=w541) -> ("error out"=w543:errorcluster, "client handle out"=w542:T8)  [unwired: 7 in]
        n226 = call "is_paused.vi"("url"=w538, "error in (no error)"=w543, "client handle"=w542) -> ("error out"=w549:errorcluster, "paused"=w545:bool, "client handle out"=w550:T8)  [unwired: 6 in]
        n227 = case shown="False" w545 {
          tunnel: w548 -> [_ w558]
          tunnel: w539 -> [w551 w560]
          tunnel: w538 -> [_ w563]
          tunnel: w549 -> [w552 w565]
          tunnel: w550 -> [w553 w564]
          tunnel: [w551 w556] -> w544
          tunnel: [w553 w555] -> w547
          tunnel: [w552 w554] -> w546
          frame True {
          }
          frame False {
            n228 = Array Size(array=w558) -> (size(s)=w557:i32)
            n229 = Index Array(array=w558, index=w560) -> (element=w566:T9)
            n230 = Increment(x=w560) -> (x+1=w559:i32)
            n231 = Quotient & Remainder(x=w559, y=w557) -> (x-y*floor(x/y)=w556:i32)  [unwired: 1 out]
            n232 = call "send_angles.vi"("url"=w563, "error in (no error)"=w565, "angles and speed"=w566, "client handle"=w564) -> ("error out"=w561:errorcluster, "client handle out"=w562:T8)  [unwired: 6 in]
            n233 = while {
              tunnel: w563 -> [w572]
              tunnel: w562 -> [w571]
              tunnel: w561 -> [w570]
              tunnel: [w568] -> w555
              tunnel: [w567] -> w554
              stop <- w569 continue-if-true
              n234 = call "is_moving.vi"("string"=w572, "error in (no error)"=w570, "client handle"=w571) -> ("error out"=w567:errorcluster, "moving"=w569:bool, "client handle out"=w568:T8)  [unwired: 6 in]
            }
          }
        }
      }
    }
  }
  n235 = call <vilib>:"CloseHandle.vi"("client handle"=w6, "error in (no error)"=w4) -> ()  [unwired: 13 in, 1 out]
  n236 = call <vilib>:"CloseHandle.vi"("client handle"=w12, "error in (no error)"=w5) -> ()  [unwired: 13 in, 1 out]
  n237 = Close File(refnum=w34, error in=w35) -> (error out=w38:errorcluster)  [unwired: 1 out]
  n238 = Close File(refnum=w16, error in=w15) -> (error out=w22:errorcluster)  [unwired: 1 out]
  n239 = Close File(refnum=w14, error in=w13) -> (error out=w21:errorcluster)  [unwired: 1 out]
  n240 = local read "iterationsIM"() -> (→"iterationsIM":dbl)
  n241 = call <vilib>:"Simple Error Handler.vi"("error in (no error)"=w38) -> ()  [unwired: 1 in, 8 out]
  n242 = call <vilib>:"Simple Error Handler.vi"("error in (no error)"=w22) -> ()  [unwired: 1 in, 8 out]
  n243 = call <vilib>:"Simple Error Handler.vi"("error in (no error)"=w21) -> ()  [unwired: 1 in, 8 out]
  n244 = call <instrlib>:"niUSRP Close Session.vi"("session handle"=w48, "error in (no error)"=w49) -> ()  [unwired: 13 in, 1 out]
  "No. Bits LP - CH0" <- w45
  "No. Bits - CH1" <- w45
  "No. Bits HP - CH0" <- w45
